vi "progra 9.vi"() -> ()   [LabVIEW 2011]
panel:
  in  "on/off prg":bool
  out "TempMin":dbl
  out "TempMaxima":dbl
  out "TempPromedio":dbl
  in  "on/off A/C":bool
  out "A/C on":bool
  in  "TempDeseada":dbl
  out "Temperatura":i32(slide) scale=0.0..50.0
  # "El programa simula el funcionamiento de una a/c\ndonde se ingresa la temperatura deseada y cada \nvez que la temperatura deseadasea mayor a la\ntemperatura no se enciende el compresor del\na/c. pero cuando esta sea menorse enciende el \ncompresor pero esto solo puede ocurrir siempre que \nel a/c este encendido, el programa termina solo cuando \ndecidimos nosotros terminar."
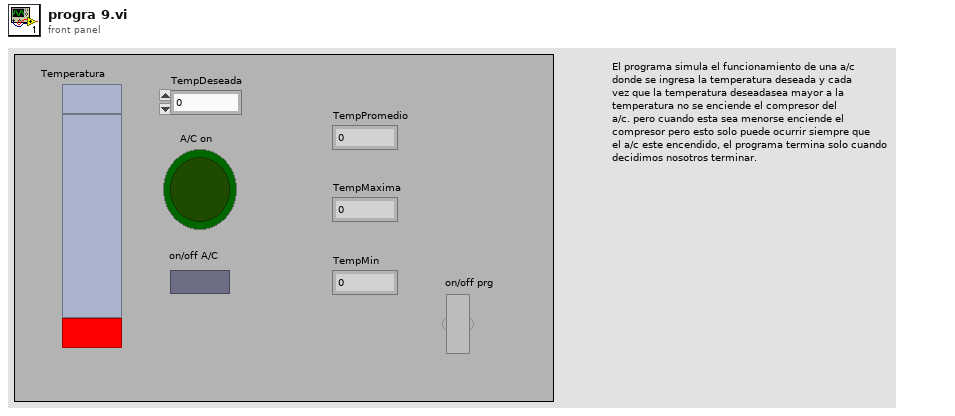
[diagram p1: front panel]
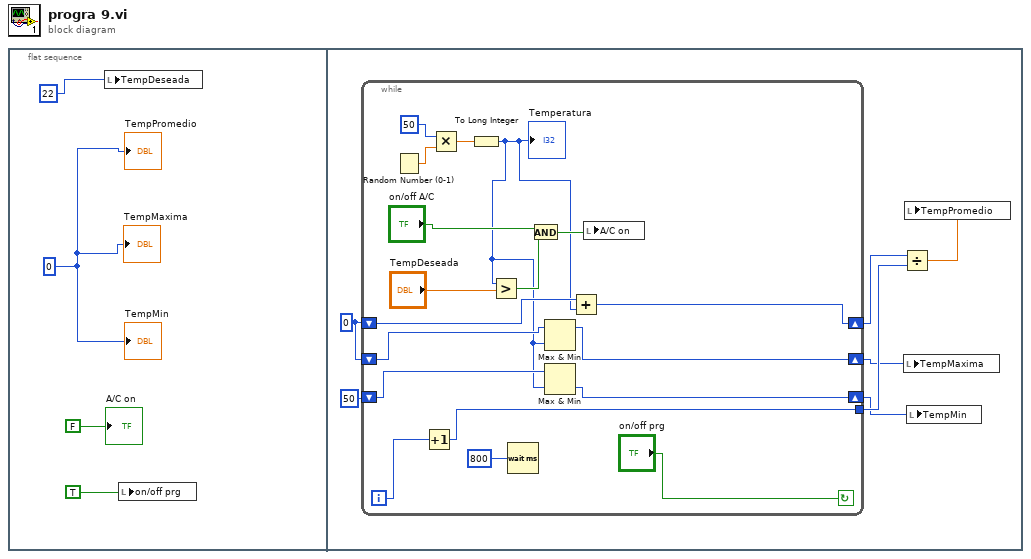
[diagram p0: block diagram]
diagram:
  n1 = flat-sequence {
    frame #0 {
      w4 = 0
      n2 = local write "TempDeseada"(22) -> ()
      n3 = local write "on/off prg"(TRUE) -> ()
      "TempPromedio" <- w4
      "TempMaxima" <- w4
      "TempMin" <- w4
      "A/C on" <- FALSE
    }
    frame #1 {
      w8 = 0
      n4 = while {
        tunnel: [w19] -> w10
        shift-right: [w17] -> w9
        shift-left: w8 -> [w18]
        shift-right: [w13] -> w7
        shift-left: w8 -> [w16]
        shift-right: [w12] -> w6
        shift-left: 50 -> [w15]
        i -> [w20]
        stop <- "on/off prg" continue-if-true
        n5 = Random Number (0-1)() -> (number: 0 to 1=w26:dbl)
        n6 = Increment(x=w20) -> (x+1=w19:i32)
        n7 = Multiply(x=50, y=w26) -> (x*y=w27:dbl)
        n8 = To Long Integer(number=w27) -> (32bit integer=w14:i32)
        "Temperatura" <- w14
        n9 = Greater?(x=w14, y="TempDeseada") -> (0:w23:bool)
        n10 = Wait (ms)(milliseconds to wait=800) -> ()  [unwired: 1 out]
        n11 = And(x="on/off A/C", y=w23) -> (x .and. y?=w21:bool)
        n12 = Max & Min(x=w16, y=w14) -> (max(x,y)=w13:i32)  [unwired: 1 out]
        n13 = Max & Min(x=w15, y=w14) -> (min(x,y)=w12:i32)  [unwired: 1 out]
        n14 = Add(x=w18, y=w14) -> (x+y=w17:i32)
        n15 = local write "A/C on"(w21) -> ()
      }
      n16 = Divide(x=w9, y=w10) -> (x/y=w11:dbl)
      n17 = local write "TempMaxima"(w7) -> ()
      n18 = local write "TempPromedio"(w11) -> ()
      n19 = local write "TempMin"(w6) -> ()
    }
  }
